vi "GetPubUpdates.vi"(1 "XML":string) -> (0 "PubUpdate":T1)   [LabVIEW 2016]
doc: "Returns a publisher update with\n-Caller ID\n-Topic name\n-an array of Node URIs"
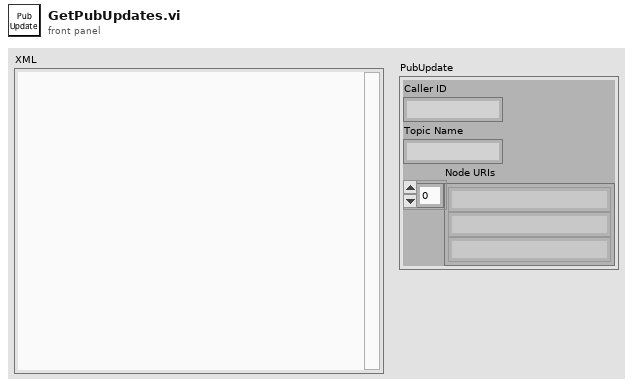
[diagram p1: front panel]
types:
  T1 = cluster{"Caller ID":string, "Topic Name":string, "Node URIs":string[]}
  T2 = cluster{"Caller ID":string, "Topic Name":string, "URIs":string[]}
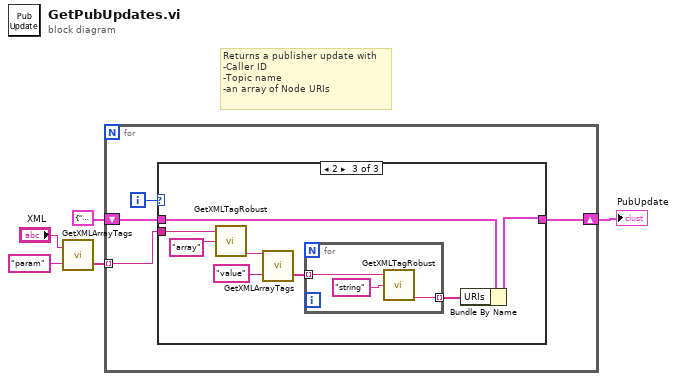
[diagram p0: block diagram]
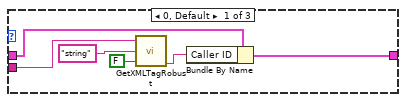
[diagram p2: hidden frame]
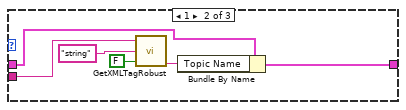
[diagram p3: hidden frame]
diagram:
  # "Returns a publisher update with\n-Caller ID\n-Topic name\n-an array of Node URIs"
  n1 = call "GetXMLArrayTags.vi"("ArrayTag"="param", "String"="XML") -> ("Array"=w5:string[])  [unwired: 1 out]
  n2 = for {
    tunnel: w5 -> [w7] mode=indexing
    shift-right: [w6] -> w2
    shift-left: T2 {"Caller ID"="", "Topic Name"="", "URIs"=[]} ("Subscriber") -> [w8]
    i -> [w9]
    n3 = case shown="2" w9 {
      tunnel: w8 -> [w13 w21 w26]
      tunnel: w7 -> [w15 w19 w24]
      tunnel: [w11 w20 w25] -> w6
      frame 0, Default {
        n4 = call "GetXMLTagRobust.vi"("Tag only? (T)"=FALSE ("Tag only?"), "Tag"="string", "String"=w15) -> ("value"=w12:string)  [unwired: 3 out]
        n5 = Bundle By Name(cluster=w13, "Caller ID"=w12) -> (w11:T2)
      }
      frame 1 {
        n6 = call "GetXMLTagRobust.vi"("Tag only? (T)"=FALSE ("Tag only?"), "Tag"="string", "String"=w19) -> ("value"=w16:string)  [unwired: 3 out]
        n7 = Bundle By Name(cluster=w21, "Topic Name"=w16) -> (w20:T2)
      }
      frame 2 {
        n8 = call "GetXMLTagRobust.vi"("Tag"="array" ("ArrayTag"), "String"=w24) -> ("value"=w22:string)  [unwired: 1 in, 3 out]
        n9 = call "GetXMLArrayTags.vi"("ArrayTag"="value", "String"=w22) -> ("Array"=w28:string[])  [unwired: 1 out]
        n10 = for {
          tunnel: w28 -> [w32] mode=indexing
          tunnel: [w30] -> w27 mode=indexing
          n11 = call "GetXMLTagRobust.vi"("Tag"="string", "String"=w32) -> ("value"=w30:string)  [unwired: 1 in, 3 out]
        }
        n12 = Bundle By Name(cluster=w26, "URIs"=w27) -> (w25:T2)
      }
    }
  }
  "PubUpdate" <- w2
